vi "databaseGF.vi"(9 "deviceDataBase in":refnum<class "deviceDataBase.lvclass">, 10 "Enum":enum16{"write", "read"}(ring)) -> (1 "deviceDataBase out":refnum<class "deviceDataBase.lvclass">)   [LabVIEW 2009, in "Tools.lvlib" / "DatabaseHelpers.lvlib"]
uses:
  DatabaseHelpers.lvlib
  deviceDataBase.lvclass
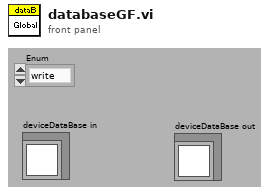
[diagram p1: front panel]
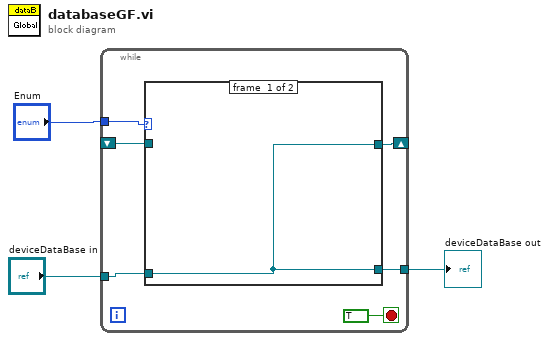
[diagram p0: block diagram]
diagram:
  n1 = while {
    tunnel: "deviceDataBase in" -> [w8]
    tunnel: "Enum" -> [w9]
    tunnel: [w4] -> w1
    shift-right: [w7] -> _
    shift-left: _ -> [w5]
    stop <- TRUE stop-if-true
    n2 = case shown="\"write\", Default" w9 {
      tunnel: w8 -> [w10 _]
      tunnel: [w10 w11] -> w7
      tunnel: w5 -> [_ w11]
      tunnel: [w10 w11] -> w4
      frame #0 {
      }
      frame #1 {
      }
    }
  }
  "deviceDataBase out" <- w1
